vi "Global_Data Out.vi"() -> ()   [LabVIEW 2017, in "Controller.lvlib"]
uses:
  Controller.lvlib
panel:
  out "Button Board Joystick":dbl[](array[numeric])
  out "Button Board":bool[](array[boolean])
  out "HW_Joystick_POVs":i16[](array[numeric])
  out "HW_Joystick_Buttons":bool[](array[boolean])
  out "HW_Joystick_Axes":dbl[](array[numeric])
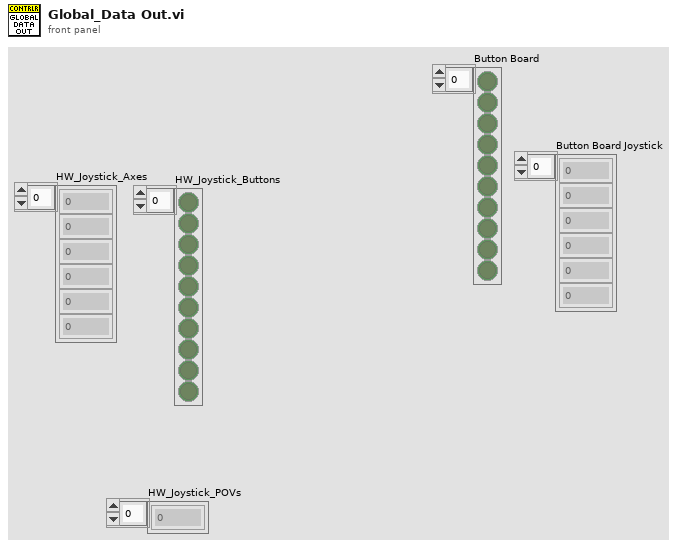
[diagram p1: front panel]
diagram:
